vi "LV86_Save JPG.vi"(2 "Path to file":path, 3 "Image":T1 {"Dialogs" format="%.0b"}) -> (1 "Image":T1 {"Dialogs" format="%.0b"})   [LabVIEW 2009]
doc: "This VI saves an image to a JPEG file."
uses:
  QT_Image.ctl
  QT_Selector.ctl
  QT_Compression.ctl
  QT_File.ctl
  QT_Private.ctl
panel:
  in  "Format":u16(ring)=1 items=["BMP", "JPEG", "MacPaint", "Photoshop", "PNG", "PICT", "SG", "Targa", "TIFF"]
  in  "Compression":i32(slide)=1023 scale=0.0..1023.0 scale format="%.0x"
  out "error out":errorcluster
  out "Path":path
  # "This VI saves an image to a JPEG file."
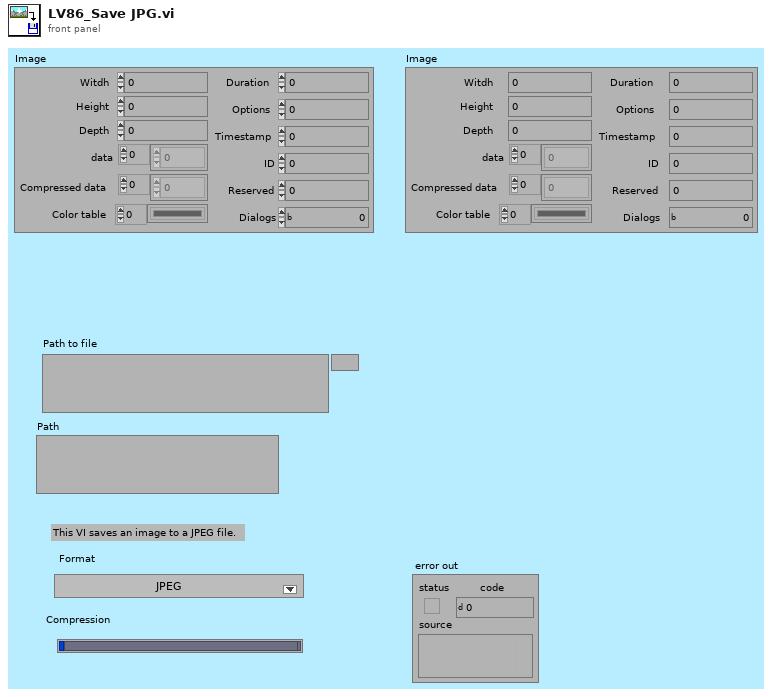
[diagram p1: front panel]
types:
  T1 = typedef "QT_Image.ctl" = cluster{"Witdh":i32, "Height":i32, "Depth":i32, "data":u8[], "Compressed data":u8[], "Color table":u32[], "Duration":i32, "Options":i32, "Timestamp":i32, "ID":i32, "Reserved":i32, "Dialogs":u32}
  T2 = typedef "QT_Selector.ctl" = enum32{"do nothing", "Get all Sources", "Get Source info", "Open Image", "Save Image to File", "Effect", "Close", "SG Grab", "Compress in Memory", "Decompress to Memory", "New Movie", "Open Movie", "Add Frame", "Get Frame", "Close Movie", "Get QT & CIN info", "SG init", "SG Close", "Open sound file", "Close sound file", "Read sound data", "Write sound data", "Import sound", "Export sound", "Add sound to movie", "Get sound from movie", "reserved", "reserved 1", "reserved 2"}
  T3 = typedef "QT_Compression.ctl" = cluster{"Compression":i32, "Format":i32, "Codec":i32, "Comp. Quality":i32, "Key Frame":i32, "Dialogs":u32}
  T4 = typedef "QT_File.ctl" = cluster{"Paths":string[], "Options":i32, "Dialogs":u32, "Reserved":i32}
  T5 = typedef "QT_Private.ctl" = cluster{"reserved 1":i32, "reserved 2":i32, "reserved 3":i32, "reserved 4":i32}
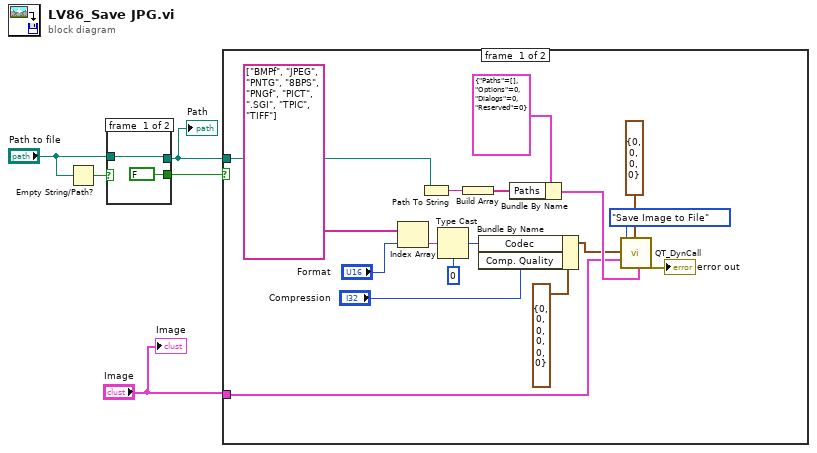
[diagram p0: block diagram]
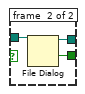
[diagram p2: hidden frame]
diagram:
  n1 = Empty String/Path?(string/path="Path to file") -> (empty?=w1:bool)
  n2 = case shown="False" w1 {
    tunnel: [FALSE ("cancelled") w10] -> w5
    tunnel: [w7 w9] -> w4
    tunnel: "Path to file" -> [w7 w8]
    frame #0 {
    }
    frame #1 {
      n3 = File Dialog(11:w8) -> (1:w10:bool, 3:w9:path)  [unwired: 1 in, 7 out]
    }
  }
  "Path" <- w4
  n4 = case shown="False" w5 {
    tunnel: w4 -> [w17 _]
    tunnel: "Image" -> [w12 _]
    frame #0 {
      n5 = Index Array(array=string[] ["BMPf", "JPEG", "PNTG", "8BPS", "PNGf", "PICT", ".SGI", "TPIC", "TIFF"], index="Format") -> (element=w24:string)
      n6 = Path To String(path=w17) -> (string=w18:string)
      n7 = Type Cast(type=0 ("Format"), x=w24) -> (*(type *) &x=w26:i32)
      n8 = Build Array(w18) -> (w27:string[])
      n9 = Bundle By Name(cluster=T3 {"Compression"=0, "Format"=0, "Codec"=0, "Comp. Quality"=0, "Key Frame"=0, "Dialogs"=0} ("Compression Settings"), "Codec"=w26, "Comp. Quality"="Compression") -> (w13:T3)
      n10 = Bundle By Name(cluster=T4 {"Paths"=[], "Options"=0, "Dialogs"=0, "Reserved"=0} ("File Settings"), "Paths"=w27) -> (w14:T4)
      n11 = call "QT_DynCall.vi"("Compression Settings"=w13, "Image in"=w12, "Selector"=QT_Selector."Save Image to File", "Private"=T5 {"reserved 1"=0, "reserved 2"=0, "reserved 3"=0, "reserved 4"=0}, "File Settings"=w14) -> ("error out"=→"error out":errorcluster)  [unwired: 7 in, 15 out]
    }
    frame #1 {
    }
  }
  "Image" <- "Image"
